vi "ListenCondensorMic.vi"() -> ()   [LabVIEW 2017]
uses:
  <vilib>/express/express analysis/Spectral/Block/exnSpectralBlock spectral measurements power poly.vi
  <vilib>/express/express analysis/Spectral/Block/exnSpectralBlock spectral measurements power DDT.vi
  <vilib>/express/express analysis/Spectral/XNode/ExpressSpectralMeasurementsBlockNode.xnode
panel:
  out "Listening":bool=TRUE
  out "Waveform Graph 3":dynamicdata(graph)
  out "Waveform Graph 2":dynamicdata(graph)
  in  "Time (sec)":dbl(knob)=25.0 min=0.0 max=60.0 step=1.0 scale=0.0..60.0 scale format="%#_2g"
  in  "Analog Acquisition  2":cluster{"Analog Fs":u32}={"Analog Fs"=10000} {"Analog Fs" format="%0.0f"}
  in  "Device Name":tag="Dev3"
  in  "File Path":path=path "C:/Users/klt8/Documents"
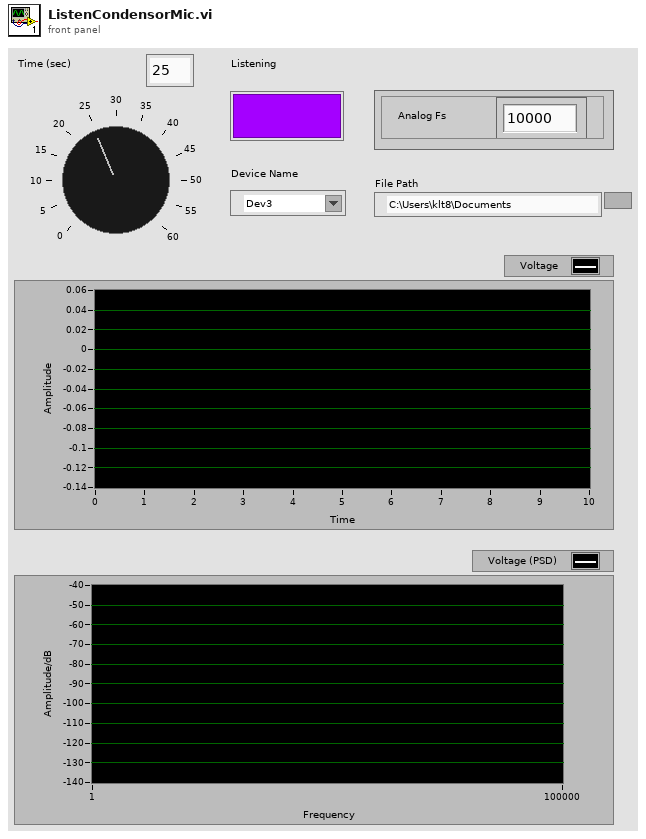
[diagram p1: front panel]
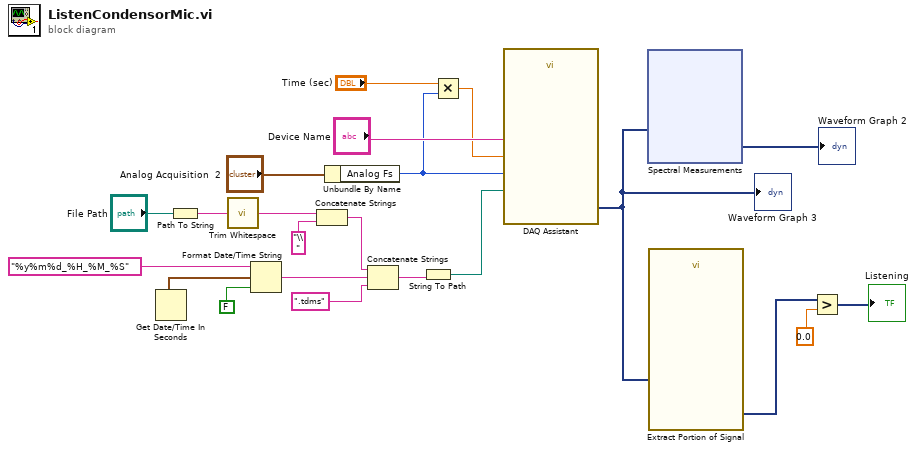
[diagram p0: block diagram]
diagram:
  n1 = Get Date/Time In Seconds() -> (seconds since 1Jan1904=w12:timestamp)
  n2 = Path To String(path="File Path") -> (string=w14:string)
  n3 = call <vilib>:"Trim Whitespace.vi"("string"=w14) -> ("trimmed string"=w15:string)  [unwired: 1 in]
  n4 = Format Date/Time String(time format string (%c)="%y%m%d_%H_%M_%S", seconds (now)=w12, UTC format=FALSE) -> (date/time string=w16:string)
  n5 = Concatenate Strings(w15, "\\" ("string")) -> (w8:string)
  n6 = Unbundle By Name("Analog Acquisition  2") -> ("Analog Fs"=w19:u32)
  n7 = Concatenate Strings(w8, w16, ".tdms" ("string")) -> (w6:string)
  n8 = String To Path(string=w6) -> (path=w5:path)
  n9 = Multiply(x="Time (sec)", y=w19) -> (x*y=w18:dbl)
  n10 = call "DAQ Assistant"("rate"=w19, "number of samples"=w18, "file path"=w5, "device name"="Device Name") -> ("data"=w4:dynamicdata)  [unwired: 13 in, 2 out]
  "Waveform Graph 3" <- w4
  n11 = xnode "Spectral Measurements"("Signals"=w4) -> ("Power Spectrum"=→"Waveform Graph 2":dynamicdata)  [unwired: 1 in, 1 out]
  n12 = call "Extract Portion of Signal"("Signals"=w4) -> ("Section"=w2:dynamicdata)  [unwired: 9 in, 1 out]
  n13 = Greater?(x=w2, y=0.0) -> (0:→"Listening":dynamicdata)
